vi "Create.vi"(7 "Direction":T1, 8 "error in (no error)":errorcluster, 9 "Custom Config Data":u8[](array[numeric]), 10 "Name":string, 11 "CIFTag in":refnum<class "CIF_NIChn_Fifo_DAQ.lvclass">) -> (0 "error out":errorcluster, 3 "CIFTag out":refnum<class "CIF_NIChn_Fifo_DAQ.lvclass">)   [LabVIEW 2021, in "CIF_NIChn_Fifo_DAQ.lvclass"]
uses:
  CIF_NIChn_Fifo_DAQ.lvclass
  CIF_NIChn_Fifo_DAQ.lvclass/CIF_NIChn_Fifo_DAQ.ctl
  CIFChannels/CIFChannels.lvclass
  CIFChannels/Typedef/Disconnect Behavior.ctl
  CIFChannels/Typedef/Channel State.ctl
  05c6e502-0377-480c-a15d-085597602460.vi
  c6f1aac1-fdda-4143-8087-f9e7d57e6170.vi
  ChannelCommon/typedef/Datatype Waveform.ctl
  ChannelCommon/ChannelCommon.lvlib
  <vilib>/CIF Foundation/CIF Utilities/Statistics/I64/Stats_I64_CIF_U.lvclass
  D:/dev/Packages/Channel_Manager/src/CIF_NIChn/NIChn/CIF_NIChn.lvclass
  D:/dev/Packages/Channel_Manager/src/CIFChannels/CIFChannels.lvclass
  D:/dev/Packages/Channel_Manager/src/CIF_NIChn/FIFO_DAQ/CIF_NIChn_Fifo_DAQ.lvclass
  CIFChannels/Typedef/Direction.ctl
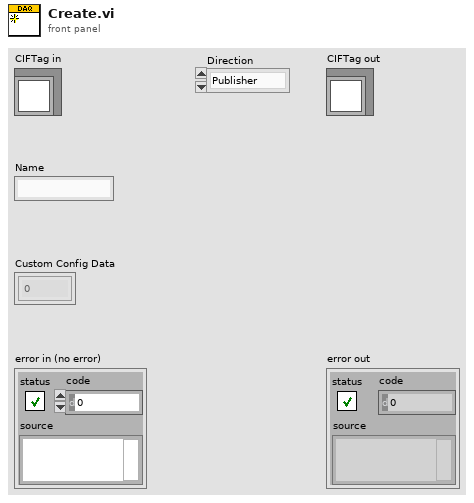
[diagram p1: front panel]
types:
  T1 = typedef "CIFChannels.lvclass/Direction.ctl" = enum16{"Publisher", "Subscriber"}
  T2 = typedef "CIFChannels.lvclass/Disconnect Behavior.ctl" = enum16{"Default value", "Last value", "Error with default"}
  T3 = typedef "ChannelCommon.lvlib/Datatype Waveform.ctl" = cluster{"measurement":dbl[], "dT":dbl, "Timestamp":i64, "Read Lock":bool}
  T4 = typedef "CIFChannels.lvclass/Channel State.ctl" = enum16{"Creating", "Disconnected", "Connecting", "Connected", "Destroyed"}
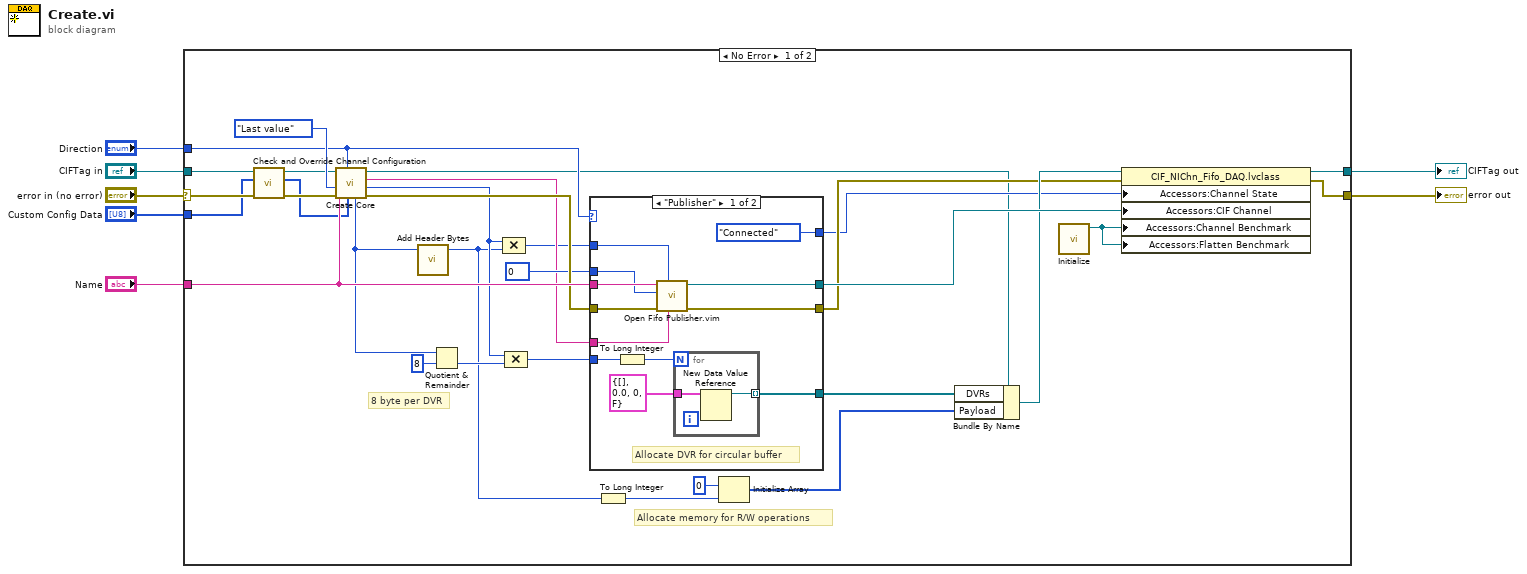
[diagram p0: block diagram]
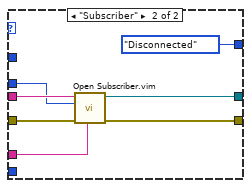
[diagram p2: hidden frame]
diagram:
  n1 = case shown="No Error" "error in (no error)" {
    selector: "error in (no error)" -> [w19 w61]
    tunnel: [w37 w61] -> w6
    tunnel: [w31 w60] -> w4
    tunnel: "CIFTag in" -> [w20 w60]
    tunnel: "Name" -> [w36 _]
    tunnel: "Direction" -> [w30 _]
    tunnel: "Custom Config Data" -> [w16 _]
    frame No Error {
      # "8 byte per DVR"
      # "Allocate memory for R/W operations"
      n2 = call-dynamic "Check and Override Channel Configuration.vi"("error in (no error)"=w19, "Custom Config Data in"=w16, "CIF_NIChn_Fifo_DAQ in"=w20) -> ("error out"=w17:errorcluster, "Custom Config Data out"=w15:u8[], "CIF_NIChn_Fifo_DAQ out"=w18:refnum<class "CIF_NIChn_Fifo_DAQ.lvclass">)  [unwired: 6 in]
      n3 = call "Create Core.vi"("Custom Config Data"=w15, "Direction"=w30, "error in (no error)"=w17, "Disconnect Behavior"=Disconnect_Behavior."Last value", "Name"=w36, "CIFChannels in"=w18) -> ("error out"=w35:errorcluster, "Messages"=w10:u64, "Channel Type"=w26:string, "CIFChannels out"=w28:refnum<class "CIF_NIChn_Fifo_DAQ.lvclass">, "Bytes/Msg"=w9:u64)  [unwired: 1 in]
      n4 = call "Add Header Bytes.vi"("Bytes/Msg"=w9) -> ("Bytes/Msg with header"=w8:u64)  [unwired: 3 in]
      n5 = Quotient & Remainder(x=w9, y=u64 8) -> (floor(x/y)=w13:u64)  [unwired: 1 out]
      n6 = Compound Arithmetic op=MULTIPLY(w10, w8) -> (w24:u64)
      n7 = Compound Arithmetic op=MULTIPLY(w10, w13) -> (w12:u64)
      n8 = case shown="\"Publisher\"" w30 {
        tunnel: w36 -> [w50 w58]
        tunnel: w35 -> [w49 w57]
        tunnel: [w45 w53] -> w34
        tunnel: [w46 w54] -> w32
        tunnel: w26 -> [w48 w56]
        tunnel: [Channel_State."Connected" ("Channel State") Channel_State."Disconnected" ("Channel State")] -> w29
        tunnel: u8 0 -> [w44 w55]
        tunnel: w24 -> [w43 _]
        tunnel: w12 -> [w40 _]
        tunnel: [w42 _] -> w22
        frame "Publisher" {
          # "Allocate DVR for circular buffer"
          n9 = To Long Integer(number=w40) -> (32bit integer=w39:i32)
          n10 = call "Open Fifo Publisher.vim"("Channel Type Description"=w48, "depth"=w43, "error in"=w49, "Input Type"=w44, "Channel Name"=w50) -> ("error out"=w46:errorcluster, "CIF Channel"=w45:refnum<k21>)  [unwired: 5 in]
          n11 = for {
            N: w39 -> [_]
            tunnel: T3 {"measurement"=[], "dT"=0.0, "Timestamp"=0, "Read Lock"=FALSE} ("Waveform Datatype") -> [w52]
            tunnel: [w51] -> w42 mode=indexing
            n12 = New Data Value Reference(data value=w52) -> (data value reference=w51:refnum<data-value>)  [unwired: 1 in, 1 out]
          }
        }
        frame "Subscriber" {
          n13 = call "Open Subscriber.vim"("Channel Type Description"=w56, "error in"=w57, "Input Type"=w55, "Channel Name"=w58) -> ("error out"=w54:errorcluster, "CIF Channel"=w53:refnum<k21>)  [unwired: 6 in]
        }
      }
      n14 = To Long Integer(number=w8) -> (32bit integer=w11:i32)
      n15 = Initialize Array(u8 0 ("Numeric"), w11) -> (w23:u8[])
      n16 = Bundle By Name(cluster=w28, "DVRs"=w22, "Payload"=w23) -> (w33:refnum<class "CIF_NIChn_Fifo_DAQ.lvclass">)
      n17 = call <vilib>:"Initialize.vi"() -> ("Stats_I64_CIF_U out"=w21:refnum<class "Stats_I64_CIF_U.lvclass">)  [unwired: 10 in, 1 out]
      n18 = property class="CIF_NIChn_Fifo_DAQ.lvclass"(reference=w33, error in=w32, "Accessors:Channel State"=w29, "Accessors:CIF Channel"=w34, "Accessors:Channel Benchmark"=w21, "Accessors:Flatten Benchmark"=w21) -> (reference out=w31:refnum<class "CIF_NIChn_Fifo_DAQ.lvclass">, error out=w37:errorcluster)
    }
    frame Error {
    }
  }
  "error out" <- w6
  "CIFTag out" <- w4
